vi "calcStuff.vi"(9 "VRefn":dbl, 10 "VRefp":dbl, 11 "Data":i32[](array[numeric])) -> (2 "stepSize(V)":dbl format="%#.20f", 3 "nOfSteps":i32)   [LabVIEW 2014]
panel:
  in  "start":i32 format="%032b"
  out "nextVolt":i32 format="%032b"
  out "-stepSize":i32 format="%032b"
  in  "stepSize":i32 format="%032b"
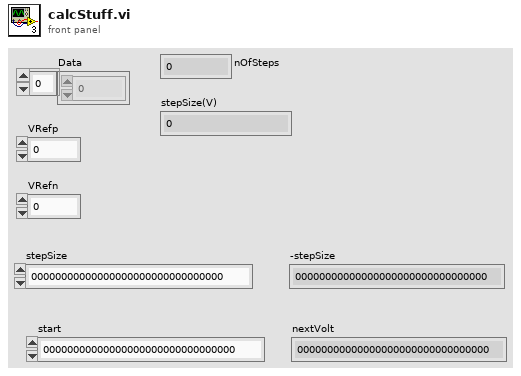
[diagram p1: front panel]
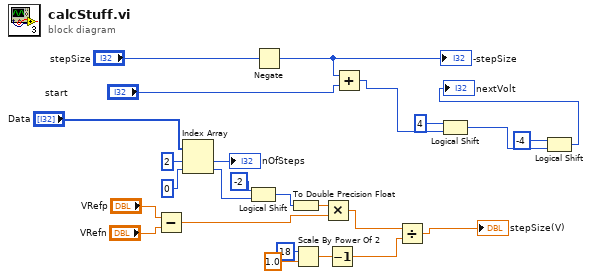
[diagram p0: block diagram]
diagram:
  n1 = Subtract(x="VRefp", y="VRefn") -> (x-y=w16:dbl)
  n2 = Index Array(array="Data", index #1=2 ("index"), index #2=0 ("index")) -> (element #1=→"nOfSteps":i32, element #2=w13:i32)
  n3 = Logical Shift(y=i16 -2, x=w13) -> (x << y=w15:i32)
  n4 = Negate(x="stepSize") -> (-x=w6:i32)
  "-stepSize" <- w6
  n5 = To Double Precision Float(number=w15) -> (double precision float=w17:dbl)
  n6 = Scale By Power Of 2(n=i16 18, x=1.0) -> (x*2^n=w20:dbl)
  n7 = Multiply(x=w17, y=w16) -> (x*y=w21:dbl)
  n8 = Decrement(x=w20) -> (x-1=w22:dbl)
  n9 = Add(x=w6, y="start") -> (x+y=w2:i32)
  n10 = Divide(x=w21, y=w22) -> (x/y=→"stepSize(V)":dbl)
  n11 = Logical Shift(y=i16 4, x=w2) -> (x << y=w3:i32)
  n12 = Logical Shift(y=i16 -4, x=w3) -> (x << y=→"nextVolt":i32)
